vi "Periodic Tasks.vi"(8 "error in":errorcluster) -> ()   [LabVIEW 2015]
doc: "This VI runs in parallel to other tasks. It can contain as many user-defined periodic loops as you need. These can carry out PID or other sorts of timed response."
uses:
  <vilib>/Rock Robotics/WPI/Utilities/WPI_GetSetVariantRefNum.vi
  Robot Global Data.vi
  <vilib>/Rock Robotics/Network Tables/SD Write Number.vi
  <vilib>/Rock Robotics/Network Tables/SD Write Boolean.vi
  <vilib>/Rock Robotics/Network Tables/NT Read Numeric Array.vi
  <vilib>/Rock Robotics/Network Tables/SD Write Numeric Array.vi
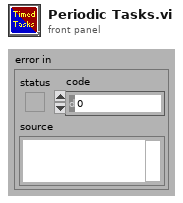
[diagram p1: front panel]
types:
  T1 = typedef "WPI_JoystickDevRef.ctl" = cluster{"Device":T2}
  T2 = typedef "WPI_JoystickDeviceEnum.ctl" = enum16{"USB 0", "USB 1", "USB 2", "USB 3", "USB 4", "USB 5"}
  T3 = cluster{"Axes[0]":dbl, "Axes[1]":dbl, "Axes[2]":dbl, "Axes[3]":dbl, "Axes[4]":dbl, "Axes[5]":dbl, "Axes[6]":dbl, "Axes[7]":dbl, "Axes[8]":dbl}
  T4 = cluster{"Buttons[0]":bool, "Buttons[1]":bool, "Buttons[2]":bool, "Buttons[3]":bool, "Buttons[4]":bool, "Buttons[5]":bool, "Buttons[6]":bool, "Buttons[7]":bool, "Buttons[8]":bool}
  T5 = typedef "WPI_EncoderDevRef.ctl" = cluster{"DevStatus":errorcluster, "EncoderIndex":T6, "CounterIndex":T7, "DistancePerCount":dbl, "Decoding Type":T8}
  T6 = typedef "FPGA_EncoderIdx.ctl" = enum8{"Enc 0", "Enc 1", "Enc 2", "Enc 3", "Enc 4", "Enc 5", "Enc 6", "Enc 7", "Invalid"}
  T7 = typedef "FPGA_CounterCtrSystemIndex.ctl" = enum8{"Ctr 0", "Ctr 1", "Ctr 2", "Ctr 3", "Ctr 4", "Ctr 5", "Ctr 6", "Ctr 7", "Invalid"}
  T8 = typedef "WPI_EncoderType.ctl" = enum16{"1x", "2x", "4x"}
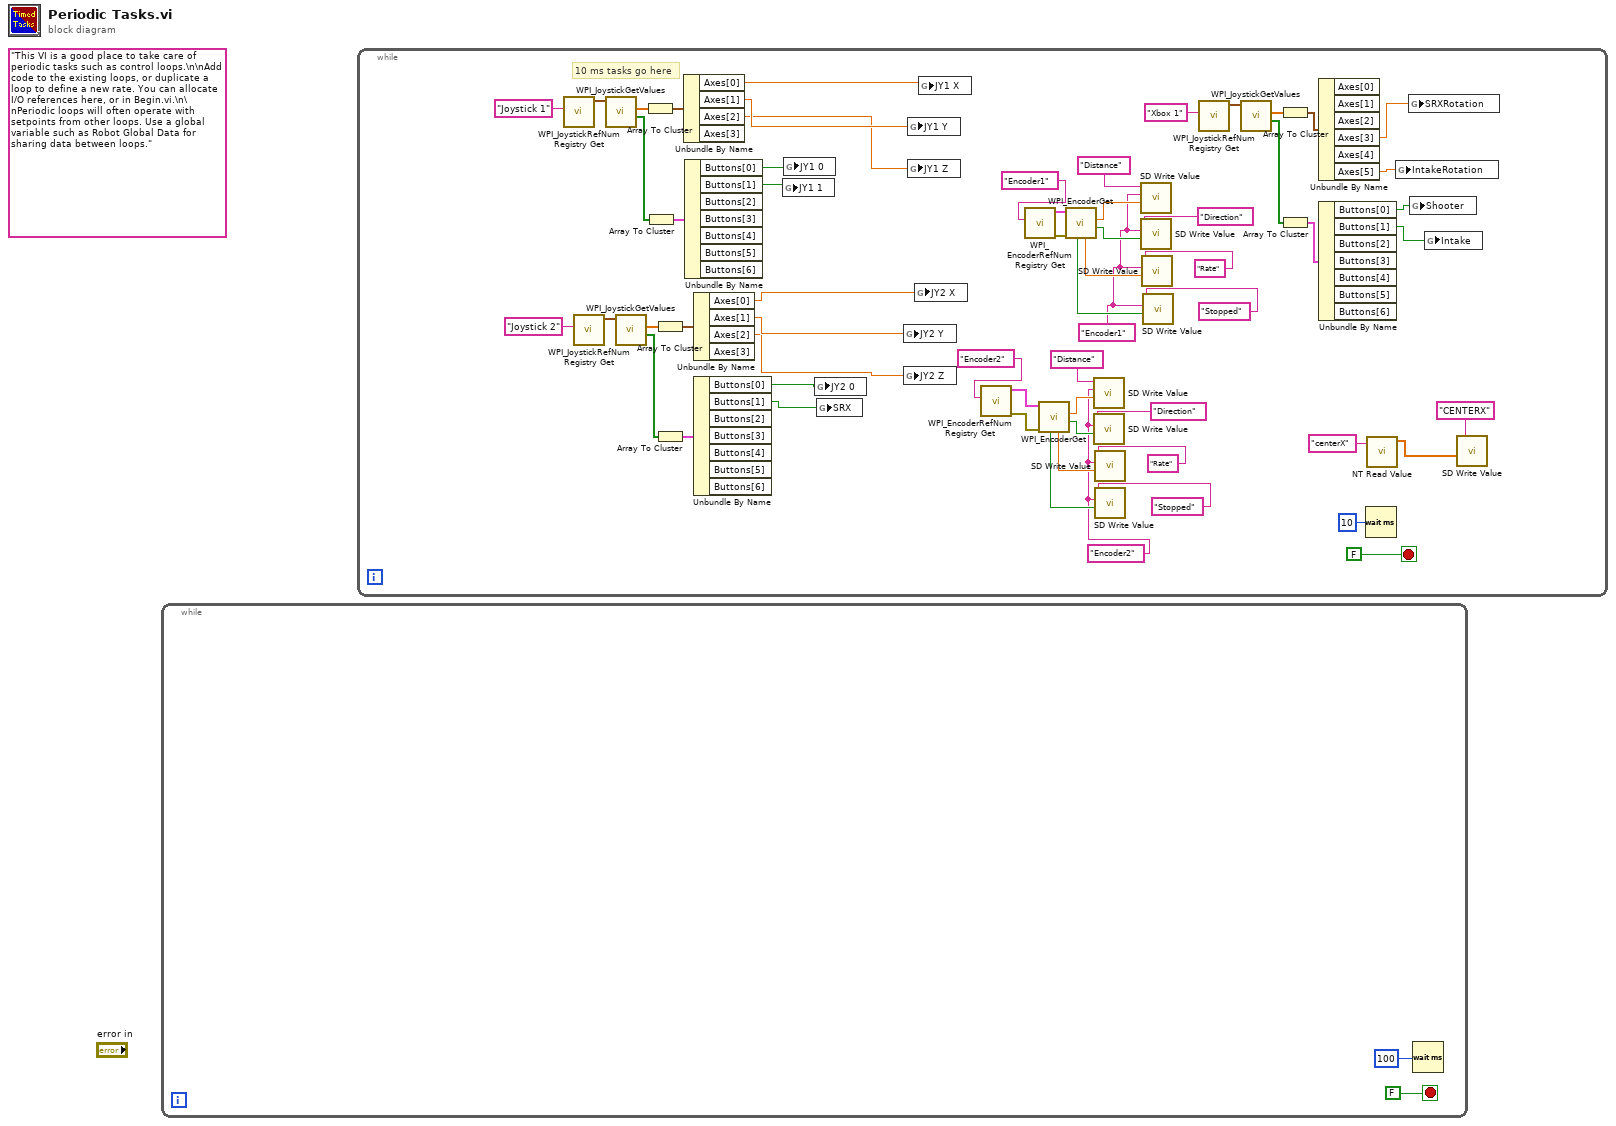
[diagram p0: block diagram]
diagram:
  (unwired) "This VI is a good place to take care of periodic tasks such as control loops.\n\nAdd code to the existing loops, or duplicate a loop to define a new rate. You can allocate I/O references here, or in Begin.vi.\n\nPeriodic loops will often operate with setpoints from other loops. Use a global variable such as Robot Global Data for sharing data between loops."
  n1 = while {
    stop <- FALSE stop-if-true
    n2 = Wait (ms)(milliseconds to wait=u32 100) -> ()  [unwired: 1 out]
  }
  n3 = while {
    stop <- FALSE stop-if-true
    w16 = "Encoder2"
    w15 = "Encoder1"
    # "10 ms tasks go here"
    n4 = call <vilib>:"WPI_JoystickRefNum Registry Get.vi"("refnum name"="Joystick 1") -> ("JoystickDevRef"=w62:T1)  [unwired: 1 in, 9 out]
    n5 = call <vilib>:"WPI_JoystickRefNum Registry Get.vi"("refnum name"="Joystick 2") -> ("JoystickDevRef"=w56:T1)  [unwired: 1 in, 9 out]
    n6 = call <vilib>:"WPI_JoystickGetValues.vi"("JoystickDevRef"=w62) -> ("Buttons"=w60:bool[], "Axes"=w59:dbl[])  [unwired: 6 in, 3 out]
    n7 = call <vilib>:"WPI_JoystickGetValues.vi"("JoystickDevRef"=w56) -> ("Buttons"=w54:bool[], "Axes"=w53:dbl[])  [unwired: 6 in, 3 out]
    n8 = Array To Cluster(array=w59) -> (cluster=w61:T3)
    n9 = Array To Cluster(array=w60) -> (cluster=w58:T4)
    n10 = Array To Cluster(array=w53) -> (cluster=w55:T3)
    n11 = Array To Cluster(array=w54) -> (cluster=w52:T4)
    n12 = Unbundle By Name(w61) -> ("Axes[0]"=w8:dbl, "Axes[1]"=w7:dbl, "Axes[2]"=w6:dbl)  [unwired: 1 out]
    n13 = Unbundle By Name(w58) -> ("Buttons[0]"=w51:bool, "Buttons[1]"=w50:bool)  [unwired: 5 out]
    n14 = Unbundle By Name(w55) -> ("Axes[0]"=w5:dbl, "Axes[1]"=w4:dbl, "Axes[2]"=w3:dbl)  [unwired: 1 out]
    n15 = Unbundle By Name(w52) -> ("Buttons[0]"=w49:bool, "Buttons[1]"=w35:bool)  [unwired: 5 out]
    n16 = global write "Robot Global Data.vi" "JY1 1"(w50) -> ()
    n17 = global write "Robot Global Data.vi" "JY1 0"(w51) -> ()
    n18 = global write "Robot Global Data.vi" "JY2 0"(w49) -> ()
    n19 = global write "Robot Global Data.vi" "SRX"(w35) -> ()
    n20 = global write "Robot Global Data.vi" "JY2 Y"(w4) -> ()
    n21 = global write "Robot Global Data.vi" "JY2 Z"(w3) -> ()
    n22 = global write "Robot Global Data.vi" "JY1 Y"(w7) -> ()
    n23 = global write "Robot Global Data.vi" "JY1 Z"(w6) -> ()
    n24 = global write "Robot Global Data.vi" "JY2 X"(w5) -> ()
    n25 = global write "Robot Global Data.vi" "JY1 X"(w8) -> ()
    n26 = call <vilib>:"WPI_EncoderRefNum Registry Get.vi"("refnum name"="Encoder2") -> ("error out"=w27:errorcluster, "EncoderDevRef"=w26:T5)  [unwired: 9 in]
    n27 = call <vilib>:"WPI_EncoderRefNum Registry Get.vi"("refnum name"="Encoder1") -> ("error out"=w48:errorcluster, "EncoderDevRef"=w47:T5)  [unwired: 9 in]
    n28 = call <vilib>:"WPI_EncoderGet.vi"("error in (no error)"=w27, "EncoderDevRef"=w26) -> ("Direction"=w23:bool, "Distance"=w24:dbl, "Rate"=w22:dbl, "Stopped"=w21:bool)  [unwired: 4 in, 2 out]
    n29 = call <vilib>:"WPI_EncoderGet.vi"("error in (no error)"=w48, "EncoderDevRef"=w47) -> ("Direction"=w44:bool, "Distance"=w45:dbl, "Rate"=w43:dbl, "Stopped"=w42:bool)  [unwired: 4 in, 2 out]
    n30 = call-poly <vilib>:"SD Write Value.vi"("Numeric"=w24, "Table Prefix"=w16, "Name"="Distance") -> ()  [unwired: 7 in, 2 out]
    n31 = call-poly <vilib>:"SD Write Value.vi"("Boolean"=w23, "Table Prefix"=w16, "Name"="Direction") -> ()  [unwired: 7 in, 2 out]
    n32 = call-poly <vilib>:"SD Write Value.vi"("Numeric"=w22, "Table Prefix"=w16, "Name"="Rate") -> ()  [unwired: 7 in, 2 out]
    n33 = call-poly <vilib>:"SD Write Value.vi"("Boolean"=w21, "Table Prefix"=w16, "Name"="Stopped") -> ()  [unwired: 7 in, 2 out]
    n34 = call-poly <vilib>:"SD Write Value.vi"("Numeric"=w45, "Table Prefix"=w15, "Name"="Distance") -> ()  [unwired: 7 in, 2 out]
    n35 = call-poly <vilib>:"SD Write Value.vi"("Boolean"=w44, "Table Prefix"=w15, "Name"="Direction") -> ()  [unwired: 7 in, 2 out]
    n36 = call-poly <vilib>:"SD Write Value.vi"("Numeric"=w43, "Table Prefix"=w15, "Name"="Rate") -> ()  [unwired: 7 in, 2 out]
    n37 = call-poly <vilib>:"SD Write Value.vi"("Boolean"=w42, "Table Prefix"=w15, "Name"="Stopped") -> ()  [unwired: 7 in, 2 out]
    n38 = call <vilib>:"WPI_JoystickRefNum Registry Get.vi"("refnum name"="Xbox 1") -> ("JoystickDevRef"=w33:T1)  [unwired: 1 in, 9 out]
    n39 = call <vilib>:"WPI_JoystickGetValues.vi"("JoystickDevRef"=w33) -> ("Buttons"=w31:bool[], "Axes"=w30:dbl[])  [unwired: 6 in, 3 out]
    n40 = Array To Cluster(array=w30) -> (cluster=w32:T3)
    n41 = Array To Cluster(array=w31) -> (cluster=w29:T4)
    n42 = Unbundle By Name(w32) -> ("Axes[3]"=w9:dbl, "Axes[5]"=w10:dbl)  [unwired: 4 out]
    n43 = Unbundle By Name(w29) -> ("Buttons[0]"=w28:bool, "Buttons[1]"=w11:bool)  [unwired: 5 out]
    n44 = Wait (ms)(milliseconds to wait=u32 10) -> ()  [unwired: 1 out]
    n45 = call-poly <vilib>:"NT Read Value.vi"("Name"="centerX") -> ("Numeric Array"=w13:dbl[])  [unwired: 9 in, 1 out]
    n46 = global write "Robot Global Data.vi" "IntakeRotation"(w10) -> ()
    n47 = global write "Robot Global Data.vi" "SRXRotation"(w9) -> ()
    n48 = global write "Robot Global Data.vi" "Shooter"(w28) -> ()
    n49 = global write "Robot Global Data.vi" "Intake"(w11) -> ()
    n50 = call-poly <vilib>:"SD Write Value.vi"("Numeric Array"=w13, "Name"="CENTERX") -> ()  [unwired: 8 in, 2 out]
  }
